vi "PROJECT_UserCredentials.vi"(8 "error in":errorcluster, 10 "Password":string, 11 "Username":string) -> (0 "error out":errorcluster, 3 "Userlevel":string)   [LabVIEW 2022 SP3, in "Project.lvlib"]
doc: "____\nHAMPEL SOFTWARE ENGINEERING v2.6.0 (2023-12-19 10:54)"
uses:
  Project.lvlib
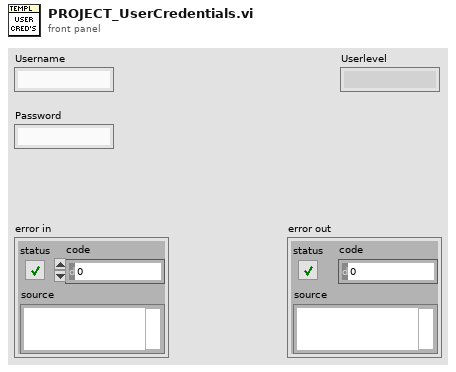
[diagram p1: front panel]
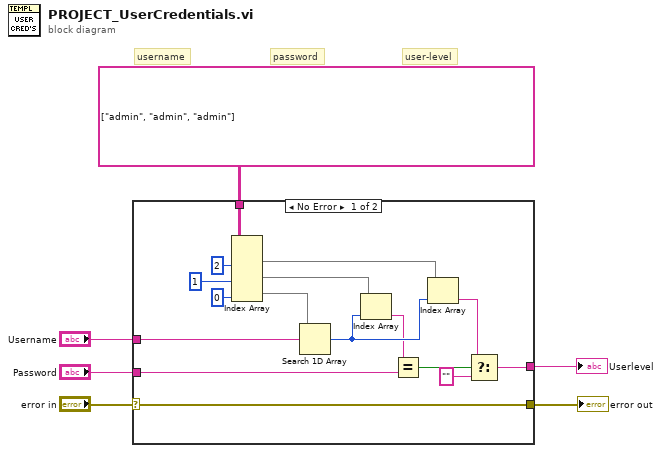
[diagram p0: block diagram]
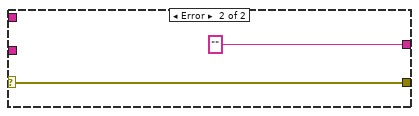
[diagram p2: hidden frame]
diagram:
  # "user-level"
  # "password"
  # "username"
  n1 = case shown="No Error" "error in" {
    selector: "error in" -> [w7 w24]
    tunnel: "Password" -> [w22 _]
    tunnel: "Username" -> [w21 _]
    tunnel: string[][] [["admin", "admin", "admin"]] ("User Table") -> [w20 _]
    tunnel: [w19 "" ("f")] -> w3
    tunnel: [w7 w24] -> w1
    frame No Error {
      n2 = Index Array(array=w20, index (col) #1=2 ("disabled index (col)"), index (col) #2=1 ("disabled index (col)"), index (col) #3=0 ("disabled index (col)")) -> (element #1=w13:string[], element #2=w14:string[], element #3=w17:string[])  [unwired: 3 in]
      n3 = Search 1D Array(1D array=w17, element=w21) -> (index of element=w12:i32)  [unwired: 1 in]
      n4 = Index Array(array=w14, index=w12) -> (element=w11:string)
      n5 = Equal?(x=w11, y=w22) -> (x = y?=w10:bool)
      n6 = Index Array(array=w13, index=w12) -> (element=w9:string)
      n7 = Select(t=w9, s=w10, f="") -> (s? t:f=w19:string)
    }
    frame Error {
    }
  }
  "Userlevel" <- w3
  "error out" <- w1
